vi "Shooter Control.vi"(11 "Time Delay Milli":dbl) -> ()   [LabVIEW 2011]
uses:
  PID Set Points.vi
  Actual RPM Global.vi
  <vilib>/addons/control/pid/pid.llb/PID (DBL).vi
  <vilib>/addons/control/pid/NI_PID_pid.lvlib
panel:
  out "Indexer RPM":cluster{dbl, dbl, dbl[]}(graph)
  out "RPM Error":dbl
  out "Encoder Speed":dbl
  in  "D":dbl
  in  "I":dbl
  out "Encoder Set Speed":dbl
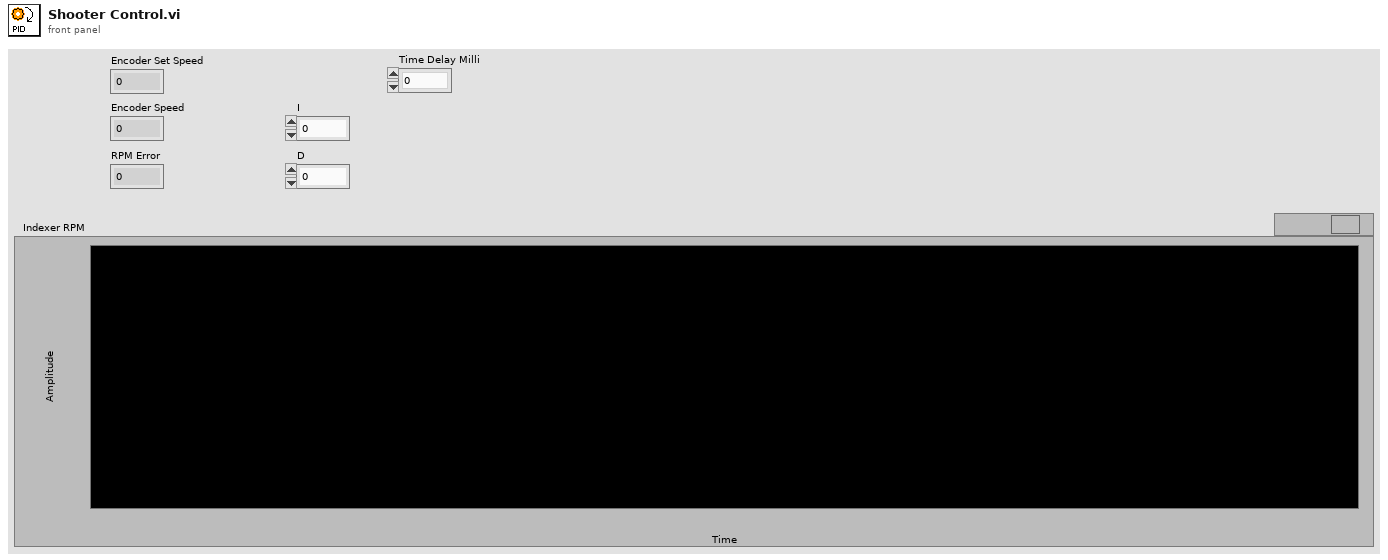
[diagram p1: front panel]
types:
  T1 = typedef "WPI_EncoderDevRef.ctl" = cluster{"DevStatus":errorcluster, "EncoderIndex":T2, "CounterIndex":T3, "DistancePerCount":dbl, "Decoding Type":T4}
  T2 = typedef "FPGA_EncoderIdx.ctl" = enum8{"Enc 0", "Enc 1", "Enc 2", "Enc 3", "Invalid"}
  T3 = typedef "FPGA_CounterCtrSystemIndex.ctl" = enum8{"Ctr 0", "Ctr 1", "Ctr 2", "Ctr 3", "Ctr 4", "Ctr 5", "Ctr 6", "Ctr 7", "Invalid"}
  T4 = typedef "WPI_EncoderType.ctl" = enum16{"1x", "2x", "4x"}
  T5 = typedef "WPI_MotorControlDeviceRef.ctl" = cluster{"DeviceStatus":errorcluster, "Type":enum16{"PWM", "CAN"}, "PWM":cluster{"Digital Module":T6, "PWM Channel":T7, "DeadBand":T8}, "CAN":cluster{"Device Number":u8, "Control Mode":T9, "Semaphore":T10, "Max Vout":dbl}, "Invert":bool, "TransformRef":T11, "InvTransformRef":T11}
  T6 = typedef "FPGA_TypedefDigitalModule.ctl" = enum16{"Digital Module 1", "Digital Module 2"}
  T7 = typedef "FPGA_DIOPWMChannel.ctl" = enum8{"PWM 1", "PWM 2", "PWM 3", "PWM 4", "PWM 5", "PWM 6", "PWM 7", "PWM 8", "PWM 9", "PWM 10", "Invalid"}
  T8 = typedef "WPI_PWMDeadband.ctl" = cluster{"Name":string, "maxPositivePwm":i32, "minPositivePwm":i32, "centerPwm":i32, "maxNegativePwm":i32, "minNegativePwm":i32, "angularRange":u16}
  T9 = typedef "WPI_CANJaguar_ControlMode.ctl" = enum8{"Percent VBus", "Current", "Speed", "Position", "Voltage"}
  T10 = typedef "Semaphore RefNum" = refnum<k1>
  T11 = typedef "WPI_PWMTransform_ConPane.ctl" = refnum<vi>
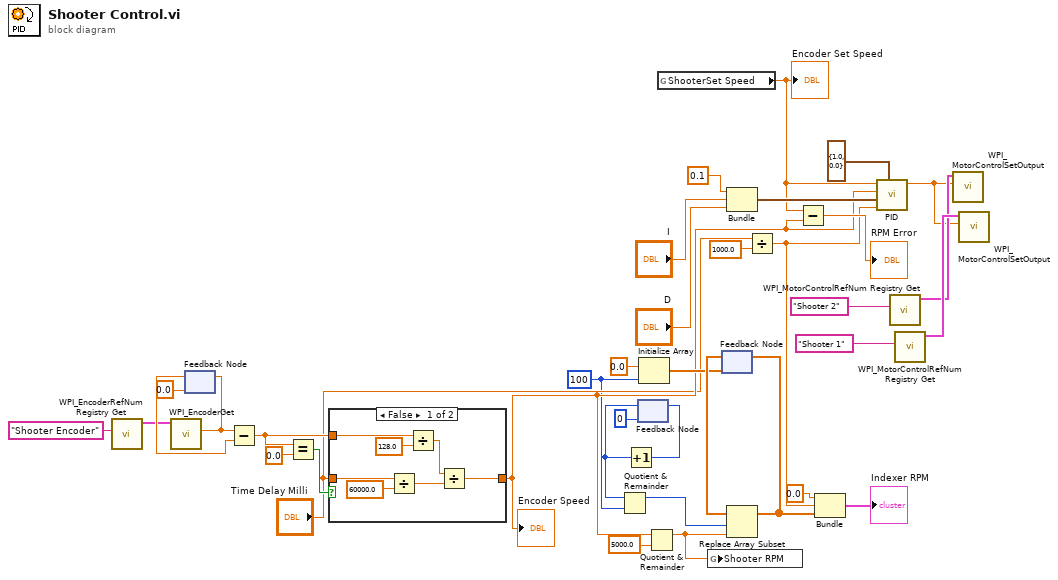
[diagram p0: block diagram]
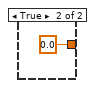
[diagram p2: hidden frame]
diagram:
  w7 = 100 ("dimension size")
  n1 = call <vilib>:"WPI_EncoderRefNum Registry Get.vi"("refnum name"="Shooter Encoder") -> ("EncoderDevRef"=w13:T1)  [unwired: 9 in, 1 out]
  n2 = call <vilib>:"WPI_EncoderGet.vi"("EncoderDevRef"=w13) -> ("Distance"=w18:dbl)  [unwired: 5 in, 5 out]
  n3 = feedback #1(0.0) -> (w21:dbl)
  n4 = feedback-in #1(w18) -> ()
  n5 = Subtract(x=w18, y=w21) -> (x-y=w15:dbl)
  n6 = Equal?(x=w15, y=0.0) -> (x = y?=w16:bool)
  n7 = case shown="False" w16 {
    tunnel: [w43 0.0] -> w12
    tunnel: w15 -> [w42 _]
    tunnel: "Time Delay Milli" -> [w40 _]
    frame False {
      n8 = Divide(x=w40, y=60000.0) -> (x/y=w38:dbl)
      n9 = Divide(x=w42, y=128.0) -> (x/y=w41:dbl)
      n10 = Divide(x=w41, y=w38) -> (x/y=w43:dbl)
    }
    frame True {
    }
  }
  "Encoder Speed" <- w12
  n11 = feedback #2(0) -> (w3:i32)
  n12 = Quotient & Remainder(x=w3, y=w7) -> (x-y*floor(x/y)=w6:i32)  [unwired: 1 out]
  n13 = Increment(x=w3) -> (x+1=w2:i32)
  n14 = feedback-in #2(w2) -> ()
  n15 = Initialize Array(0.0 ("element"), w7) -> (w23:dbl[])
  n16 = Quotient & Remainder(x=w12, y=5000.0) -> (x-y*floor(x/y)=w10:dbl)  [unwired: 1 out]
  n17 = global read "PID Set Points.vi" "ShooterSet Speed"() -> (w27:dbl)
  "Encoder Set Speed" <- w27
  n18 = global write "Actual RPM Global.vi" "Shooter RPM"(w10) -> ()
  n19 = feedback #3(w23) -> (w24:dbl[])
  n20 = Bundle(0.1, "I"="I", "D"="D") -> (w34:cluster{dbl, "I":dbl, "D":dbl})  [unwired: 1 in]
  n21 = Replace Array Subset(array=w24, new element=w10, index=w6) -> (w26:dbl[])
  n22 = feedback-in #3(w26) -> ()
  n23 = Divide(x="Time Delay Milli", y=1000.0) -> (x/y=w5:dbl)
  n24 = Subtract(x=w27, y=w12) -> (x-y=→"RPM Error":dbl)
  n25 = Bundle(0.0, w5, w26) -> (→"Indexer RPM":cluster{dbl, dbl, dbl[]})  [unwired: 1 in]
  n26 = call-poly <vilib>:"PID.vi"("output range"=cluster{"output high":dbl, "output low":dbl} {"output high"=1.0, "output low"=0.0}, "dt (s)"=w5, "PID gains"=w34, "process variable"=w12, "setpoint"=w27) -> ("output"=w29:dbl)  [unwired: 5 in, 1 out]
  n27 = call <vilib>:"WPI_MotorControlRefNum Registry Get.vi"("refnum name"="Shooter 2") -> ("MotorControlDevRef"=w30:T5)  [unwired: 9 in, 1 out]
  n28 = call <vilib>:"WPI_MotorControlRefNum Registry Get.vi"("refnum name"="Shooter 1") -> ("MotorControlDevRef"=w31:T5)  [unwired: 9 in, 1 out]
  n29 = call <vilib>:"WPI_MotorControlSetOutput.vi"("Output"=w29, "MotorControlDevRef"=w30) -> ()  [unwired: 8 in, 2 out]
  n30 = call <vilib>:"WPI_MotorControlSetOutput.vi"("Output"=w29, "MotorControlDevRef"=w31) -> ()  [unwired: 8 in, 2 out]
